vi "terminate.vi"(8 "error in (no error)":errorcluster, 11 "GenericPlugin in":refnum<class "FPGAWrapperRK110512Fiber_Spiral.lvclass">) -> (0 "error out":errorcluster, 3 "GenericPlugin out":refnum<class "FPGAWrapperRK110512Fiber_Spiral.lvclass">)   [LabVIEW 2010, in "FPGAWrapperRK110512Fiber_Spiral.lvclass"]
doc: "The dynamic dispatch version of this VI terminates the plug-in object by releasing all of its resources."
uses:
  FPGAWrapperRK110512Fiber_Spiral.lvclass
  FPGA_VI_Reference.ctl
  <vilib>/rvi/interface/nirviCloseFPGA/nirviCloseFPGA.xnode
  GenericFPGAWrapper/GenericFPGAWrapper/GenericFPGAWrapper.lvclass
  <vilib>/FPGAPlugInAG/Dynamic/niLvFpga_Close_Dynamic.vi
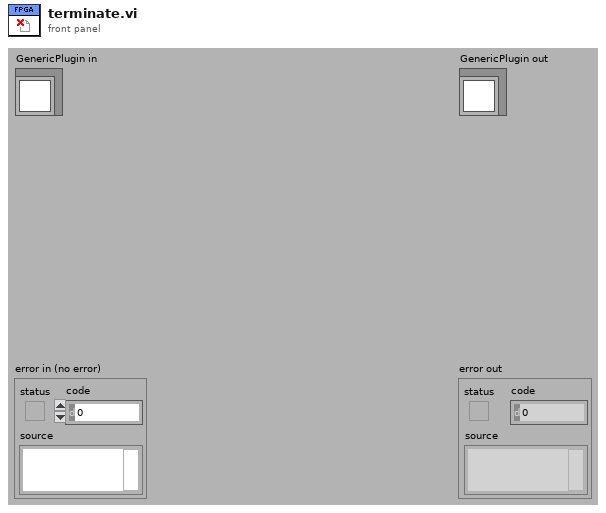
[diagram p1: front panel]
types:
  T1 = typedef "FPGAWrapperRK110512Fiber_Spiral.lvclass/FPGA_VI_Reference.ctl" = refnum<k20>
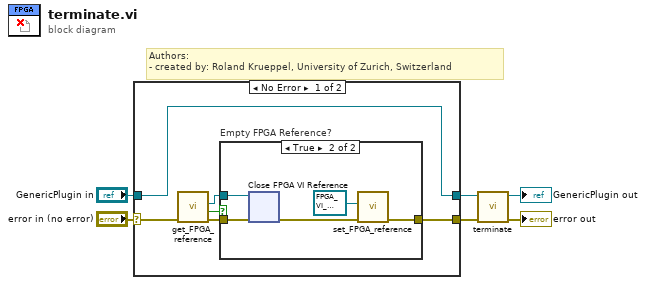
[diagram p0: block diagram]
diagram:
  # "Authors: \n- created by: Roland Krueppel, University of Zurich, Switzerland"
  n1 = case shown="No Error" "error in (no error)" {
    selector: "error in (no error)" -> [w12 w26]
    tunnel: [w8 w26] -> w3
    tunnel: [w7 w25] -> w2
    tunnel: "GenericPlugin in" -> [w7 w25]
    frame No Error {
      n2 = call "get_FPGA_reference.vi"("error in (no error)"=w12) -> ("error out"=w9:errorcluster, "is empty?"=w11:bool, "FPGA VI Reference"=w10:T1)  [unwired: 8 in]
      n3 = case "Empty FPGA Reference?" shown="True" w11 {
        tunnel: w10 -> [_ w17]
        tunnel: w9 -> [w13 w18]
        tunnel: [w13 w14] -> w8
        frame False {
        }
        frame True {
          n4 = xnode "Close FPGA VI Reference"("FPGA VI Reference In"=w17, "error in"=w18) -> ("error out"=w15:errorcluster)
          n5 = call "set_FPGA_reference.vi"("error in (no error)"=w15, "FPGA VI Reference"=T1 refnum) -> ("error out"=w14:errorcluster)  [unwired: 9 in]
        }
      }
    }
    frame Error {
    }
  }
  n6 = call-parent "terminate.vi"("error in (no error)"=w3, "GenericPlugin in"=w2) -> ("error out"=→"error out":errorcluster, "GenericPlugin out"=→"GenericPlugin out":refnum<class "FPGAWrapperRK110512Fiber_Spiral.lvclass">)  [unwired: 8 in]
